vi "Write Log.vi"(8 "error in (no error)":errorcluster, 11 "LogRotate in":refnum<class "LogRotate.lvclass">) -> (0 "error out":errorcluster, 3 "LogRotate out":refnum<class "LogRotate.lvclass">)   [LabVIEW 2021, in "Error_Manager.lvlib" / "LogRotate.lvclass"]
uses:
  LogRotate.lvclass
  LogData.ctl
panel:
  in  "LogData":T1 {"Time Stamp" format="%<%x %.3X>T"}
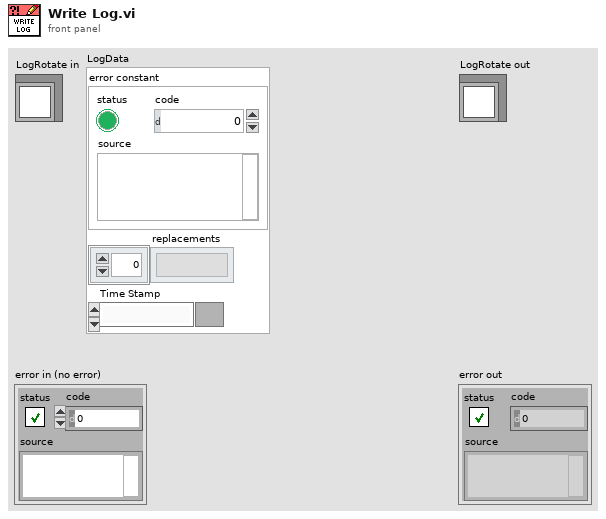
[diagram p1: front panel]
types:
  T1 = typedef "Error_Manager.lvlib/LogRotate.lvclass/LogData.ctl" = cluster{"error constant":errorcluster, "replacements":string[], "Time Stamp":timestamp}
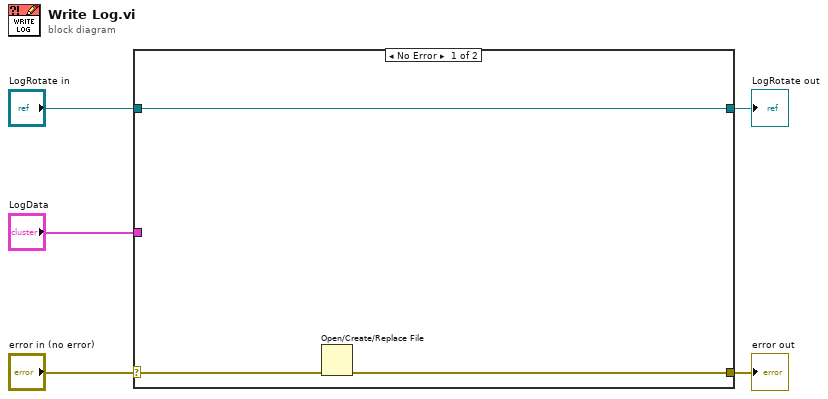
[diagram p0: block diagram]
diagram:
  n1 = case shown="No Error" "error in (no error)" {
    selector: "error in (no error)" -> [w7 w10]
    tunnel: [w6 w10] -> w4
    tunnel: [w8 w9] -> w2
    tunnel: "LogRotate in" -> [w8 w9]
    tunnel: "LogData" -> [_ _]
    frame No Error {
      n2 = Open/Create/Replace File(error in=w7) -> (error out=w6:errorcluster)  [unwired: 5 in, 2 out]
    }
    frame Error {
    }
  }
  "error out" <- w4
  "LogRotate out" <- w2
